vi "数据查询_数据查询.vi"() -> ()   [LabVIEW 2016, in "数据查询.lvlib"]
uses:
  System.Windows.Forms
  <vilib>/Utility/miscctls.llb/LVPointTypeDef.ctl
  <userlib>/_OpenG.lib/array/array.llb/Sort 2D Array (String)__ogtk.vi
  <vilib>/ptbypt/NI_PtbyPt.lvlib
panel:
  in  "数据类型":string(combo)="N"
  out "columns":string[](array[string])
  out "表格":string[][](table)
  in  "剔除异常数据":bool=TRUE
  in  "WebBrowser":refnum<k24>(container)
  in  "列表框":i32(listbox)
  in  "导出":bool
  in  "测量模式":string(combo)="全部数据"
  out "选中数据表":string
  in  "查询":bool
  in  "结束日期":string="2050/01/01"
  in  "起始日期":string="2010/01/01"
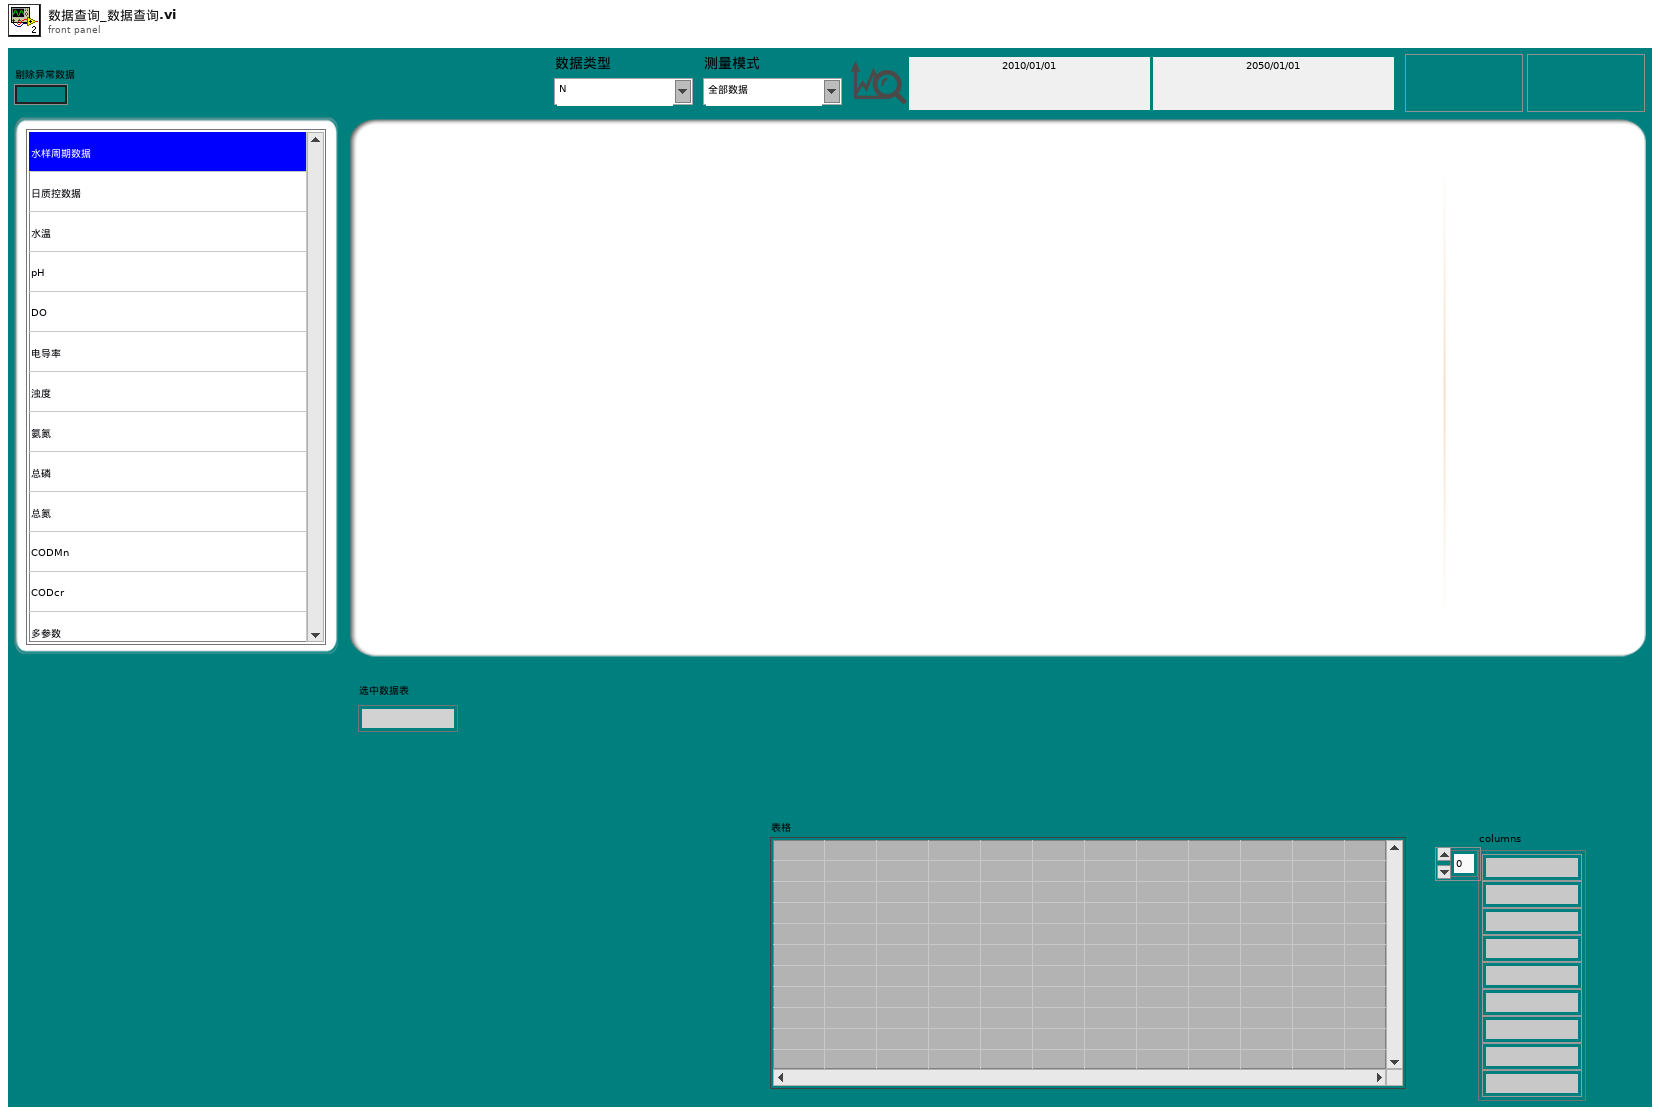
[diagram p1: front panel]
types:
  T1 = typedef "LVPointTypeDef.ctl" = cluster{"Horizontal":i16, "Vertical":i16}
  T2 = typedef "LVDateTimeRec.ctl" = cluster{"秒数的小数部分":dbl, "秒":i32, "分":i32, "时":i32, "日":i32, "月":i32, "年":i32, "天数（周）":i32, "天数（年）":i32, "DST":i32}
  T3 = typedef "数据查询菜单.xctl/数据 1.ctl" = enum32{"数据查询", "仪器数据", "仪器日志", "报警信息", "校准日志"}
  T4 = enum8{"Enabled", "Disabled", "Disabled and Grayed Out"}
  T5 = typedef "数据库类型.ctl" = enum16{"Access", "SQLite"}
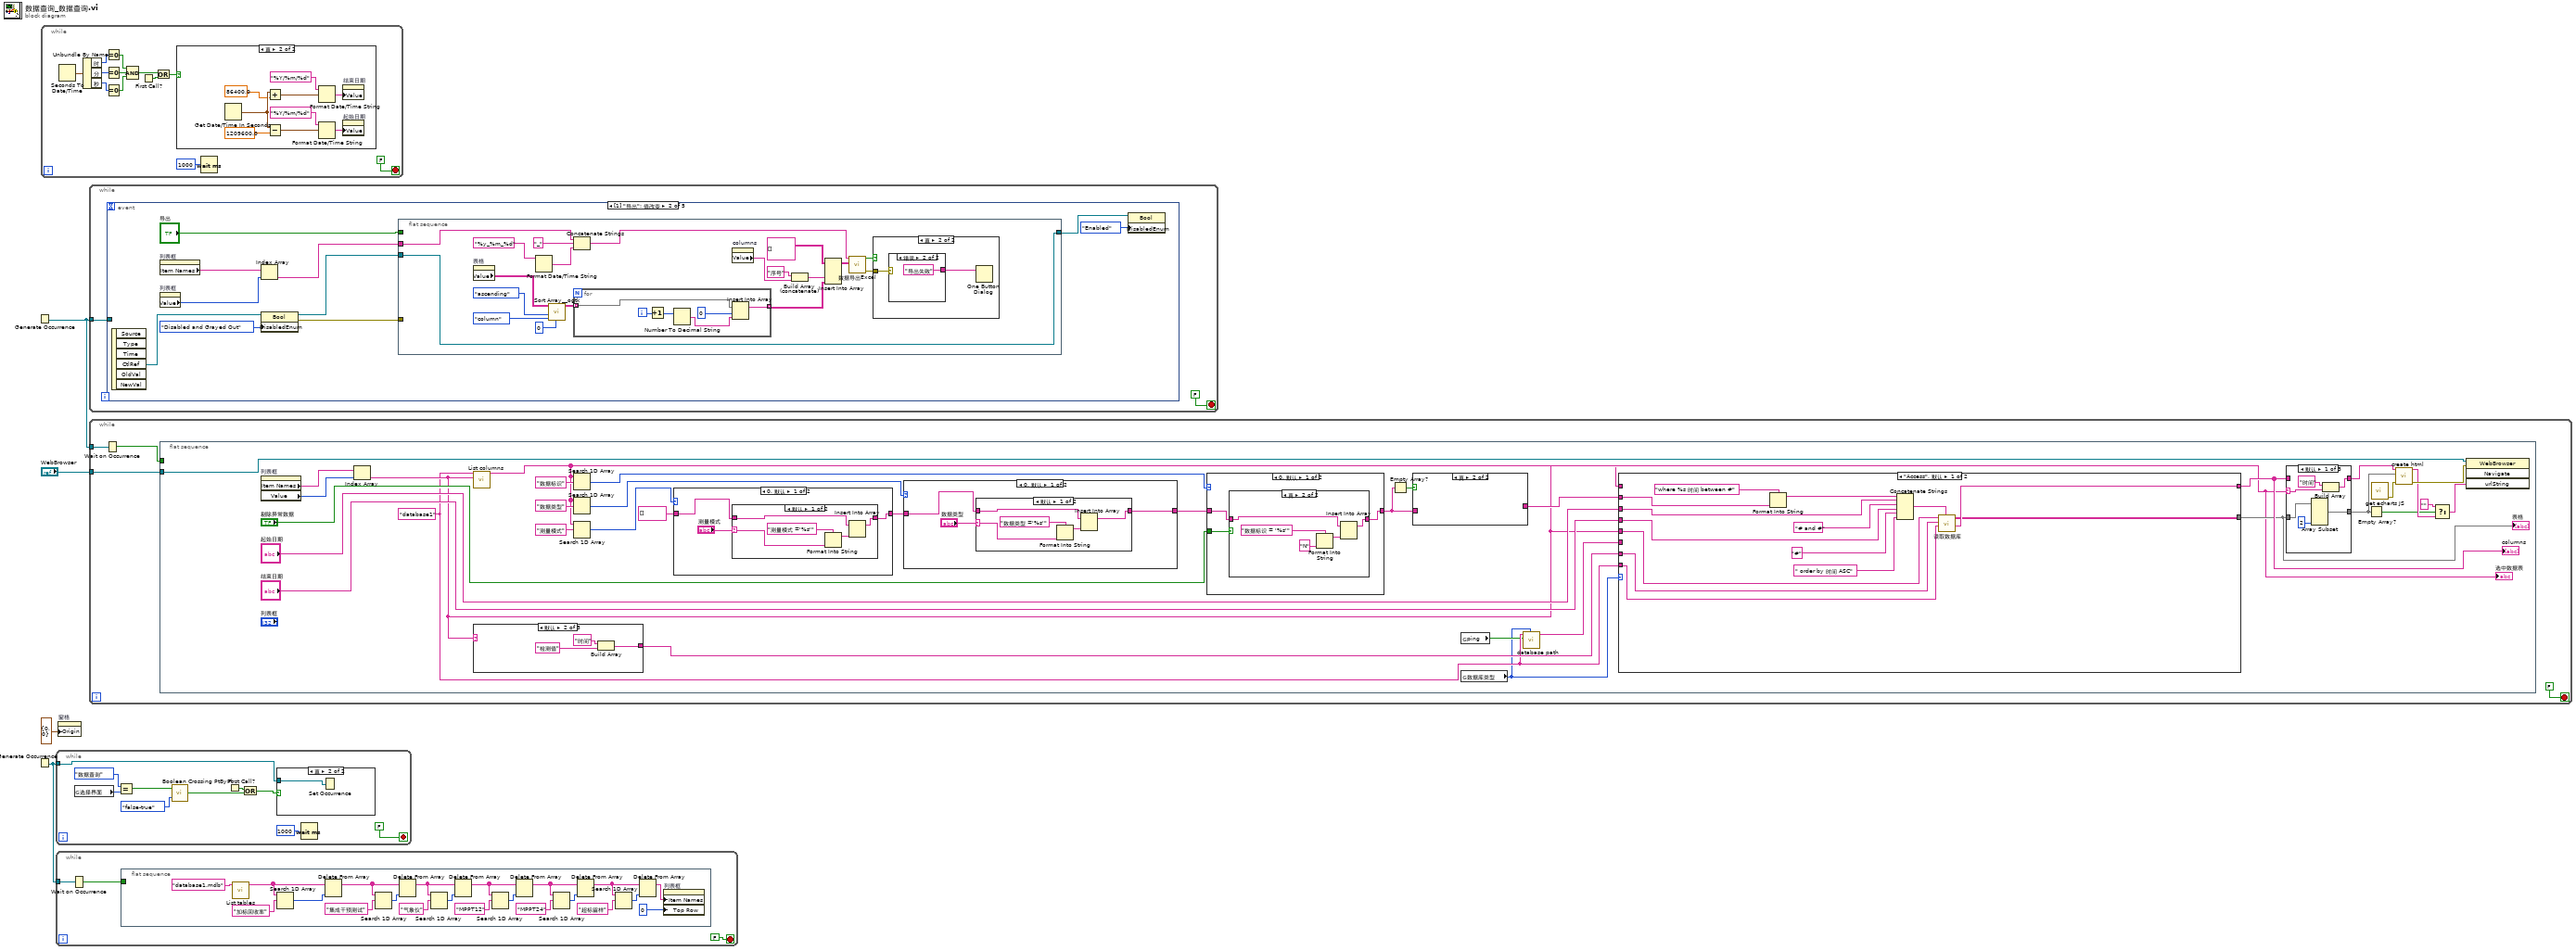
[diagram p0: block diagram]
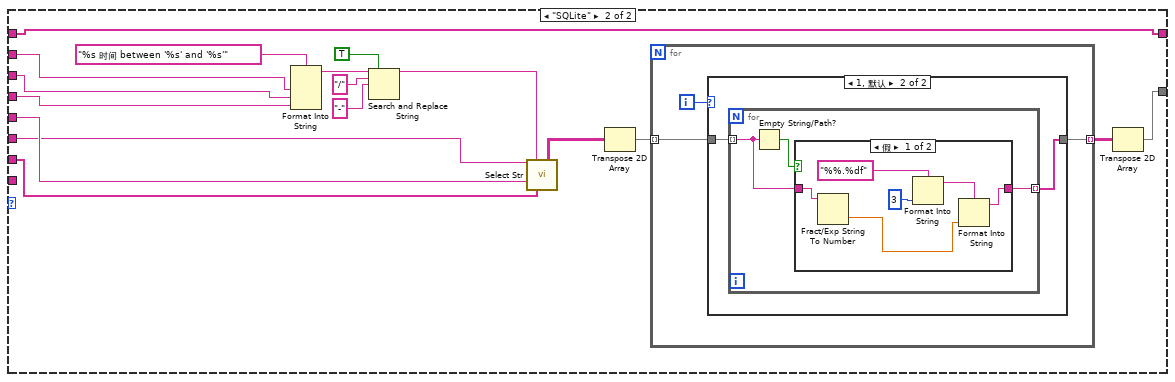
[diagram p3: hidden frame]
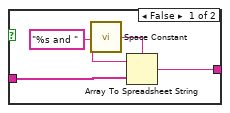
[diagram p6: hidden frame]
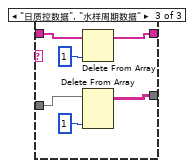
[diagram p14: hidden frame]
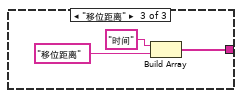
[diagram p16: hidden frame]
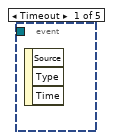
[diagram p18: hidden frame]
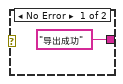
[diagram p20: hidden frame]
diagram:
  n1 = Generate Occurrence() -> (w3:refnum<k4>)
  n2 = Generate Occurrence() -> (w1:refnum<k4>)
  n3 = while {
    stop <- FALSE stop-if-true
    n4 = Seconds To Date/Time() -> (date time rec=w16:T2)  [unwired: 2 in]
    n5 = Unbundle By Name(w16) -> ("时"=w15:i32, "分"=w14:i32, "秒"=w13:i32)
    n6 = Equal To 0?(x=w15) -> (x = 0?=w12:bool)
    n7 = Equal To 0?(x=w14) -> (x = 0?=w11:bool)
    n8 = Equal To 0?(x=w13) -> (x = 0?=w10:bool)
    n9 = Compound Arithmetic op=AND ("复合运算")(w12, w11, w10) -> (w7:bool)
    n10 = First Call?() -> (First Call?: T/F=w5:bool)
    n11 = Or(x=w7, y=w5) -> (x .or. y?=w6:bool)
    n12 = case shown="真" w6 {
      frame False {
      }
      frame True {
        n13 = Get Date/Time In Seconds() -> (seconds since 1Jan1904=w21:timestamp)
        n14 = Add(x=w21, y=86400.0) -> (x+y=w19:timestamp)
        n15 = Subtract(x=w21, y=1209600.0) -> (x-y=w22:timestamp)
        n16 = Format Date/Time String(time format string (%c)="%Y/%m/%d" ("时间格式字符串(%c)"), seconds (now)=w19) -> (date/time string=w18:string)  [unwired: 1 in]
        n17 = Format Date/Time String(time format string (%c)="%Y/%m/%d" ("时间格式字符串(%c)"), seconds (now)=w22) -> (date/time string=w24:string)  [unwired: 1 in]
        n18 = property on="结束日期" class="Str"("Value"=w18) -> ()  [unwired: 2 in, 2 out]
        n19 = property on="起始日期" class="Str"("Value"=w24) -> ()  [unwired: 2 in, 2 out]
      }
    }
    n20 = Wait (ms)(milliseconds to wait=u32 1000 ("等待时间（毫秒）")) -> ()  [unwired: 1 out]
  }
  n21 = while {
    tunnel: w1 -> [w33]
    stop <- FALSE stop-if-true
    n22 = global read "全局变量.vi" "选择界面"() -> (w32:T3)
    n23 = Equal?(x=数据_1."数据查询", y=w32) -> (x = y?=w30:bool)
    n24 = call <vilib>:"Boolean Crossing PtByPt.vi"("direction"=enum16{"either", "false-true", "true-false"}."false-true", "input"=w30) -> ("crossing"=w28:bool)  [unwired: 1 in]
    n25 = First Call?() -> (First Call?: T/F=w26:bool)
    n26 = Or(x=w26, y=w28) -> (x .or. y?=w27:bool)
    n27 = case shown="真" w27 {
      tunnel: w33 -> [_ w36]
      frame False {
      }
      frame True {
        n28 = Set Occurrence(w36) -> ()
      }
    }
    n29 = Wait (ms)(milliseconds to wait=u32 1000 ("等待时间（毫秒）")) -> ()  [unwired: 1 out]
  }
  n30 = while {
    tunnel: w1 -> [w38]
    stop <- FALSE stop-if-true
    n31 = Wait on Occurrence(2:w38) -> (0:w37:bool)  [unwired: 2 in]
    n32 = flat-sequence {
      tunnel: w37 -> [_]
      frame #0 {
        n33 = call "List tables.vi"("database"="database1.mdb") -> ("tables"=w44:string[])  [unwired: 9 in, 1 out]
        n34 = Search 1D Array(1D array=w44, element="加标回收率" ("元素")) -> (index of element=w45:i32)  [unwired: 1 in]
        n35 = Delete From Array(array=w44, index=w45) -> (array with subset deleted=w47:string[])  [unwired: 1 in, 1 out]
        n36 = Search 1D Array(1D array=w47, element="集成干预测试" ("元素")) -> (index of element=w46:i32)  [unwired: 1 in]
        n37 = Delete From Array(array=w47, index=w46) -> (array with subset deleted=w50:string[])  [unwired: 1 in, 1 out]
        n38 = Search 1D Array(1D array=w50, element="气象仪" ("元素")) -> (index of element=w48:i32)  [unwired: 1 in]
        n39 = Delete From Array(array=w50, index=w48) -> (array with subset deleted=w53:string[])  [unwired: 1 in, 1 out]
        n40 = Search 1D Array(1D array=w53, element="MPPT12" ("元素")) -> (index of element=w52:i32)  [unwired: 1 in]
        n41 = Delete From Array(array=w53, index=w52) -> (array with subset deleted=w56:string[])  [unwired: 1 in, 1 out]
        n42 = Search 1D Array(1D array=w56, element="MPPT24" ("元素")) -> (index of element=w54:i32)  [unwired: 1 in]
        n43 = Delete From Array(array=w56, index=w54) -> (array with subset deleted=w57:string[])  [unwired: 1 in, 1 out]
        n44 = Search 1D Array(1D array=w57, element="超标留样" ("元素")) -> (index of element=w59:i32)  [unwired: 1 in]
        n45 = Delete From Array(array=w57, index=w59) -> (array with subset deleted=w60:string[])  [unwired: 1 in, 1 out]
        n46 = property on="列表框" class="LstBox (严格)"("Item Names"=w60, "Top Row"=0 ("顶行")) -> ()  [unwired: 2 in, 2 out]
      }
    }
  }
  n47 = property on="窗格" class="Pane"("Origin"=T1 {"Horizontal"=0, "Vertical"=0} ("原点")) -> ()  [unwired: 2 in, 2 out]
  n48 = while {
    tunnel: w3 -> [w61]
    stop <- FALSE stop-if-true
    n49 = event shown="[1] \"导出\": 值改变" {
      selector: _ -> [_ _ _ _ _]
      dyn-events: _ -> [_ _ _ _ _]
      timeout: _ -> [_ _ _ _ _]
      tunnel: w61 -> [_ _ _ w106 w107]
      event Timeout {
        n50 = event-data() -> ()  [unwired: 1 in, 3 out]
      }
      event "导出": Value Change {
        n51 = event-data() -> ("CtlRef"=w72:refnum<vi>)  [unwired: 1 in, 5 out]
        n52 = property on="列表框" class="LstBox (严格)"() -> ("Item Names"=w65:string[])  [unwired: 2 in, 2 out]
        n53 = property on="列表框" class="LstBox (严格)"() -> ("Value"=w64:i32)  [unwired: 2 in, 2 out]
        n54 = Index Array(array=w65, index=w64) -> (element=w63:string)
        n55 = property class="Bool"(reference=w72, "DisabledEnum"=T4."Disabled and Grayed Out" ("禁用")) -> (reference out=w69:refnum<vi>, error out=w70:errorcluster)  [unwired: 1 in]
        n56 = flat-sequence {
          tunnel: w70 -> [_]
          tunnel: [w88] -> w68
          tunnel: w69 -> [w88]
          tunnel: "导出" -> [_]
          tunnel: w63 -> [w78]
          frame #0 {
            n57 = property on="表格" class="Tbl (严格)"() -> ("Value"=w74:string[][])  [unwired: 2 in, 2 out]
            n58 = Format Date/Time String(time format string (%c)="%y_%m_%d" ("时间格式字符串(%c)")) -> (date/time string=w85:string)  [unwired: 2 in]
            n59 = call-poly <userlib>:"Sort Array__ogtk.vi"("Column/Row to Sort By"=u32 0, "Sort By in"=enum16{"row", "column"}."column", "Order"=enum16{"ascending", "descending"}."ascending", "Array in"=w74) -> ("Sorted Array out"=w82:string[][])  [unwired: 4 in, 3 out]
            n60 = Concatenate Strings(w78, "_" ("字符串"), w85) -> (w83:string)
            n61 = for {
              tunnel: w82 -> [w100] mode=indexing
              tunnel: [w99] -> w75 mode=indexing
              i -> [w101]
              n62 = Increment(x=w101) -> (x+1=w97:i32)
              n63 = Number To Decimal String(number=w97) -> (decimal integer string=w96:string)  [unwired: 1 in]
              n64 = Insert Into Array(array=w100, index=0 ("索引"), new element=w96) -> (w99:string[])
            }
            n65 = property on="columns" class="Arr (严格)"() -> ("Value"=w73:string[])  [unwired: 2 in, 2 out]
            n66 = Build Array (concatenate)("序号" ("新元素/子数组"), w73) -> (w76:string[])
            n67 = Insert Into Array(array=string[][] [], new element #1=w76, new element #2=w75) -> (w81:string[][])  [unwired: 2 in]
            n68 = call "数据导出Excel.vi"("text data"=w81, "default name"=w83) -> ("error out"=w80:errorcluster, "布尔"=w79:bool)  [unwired: 8 in]
            n69 = case shown="真" w79 {
              tunnel: w80 -> [_ w93]
              frame False {
              }
              frame True {
                n70 = case shown="错误" w93 {
                  tunnel: ["导出成功" ("消息") "导出失败" ("消息")] -> w92
                  frame No Error {
                  }
                  frame Error {
                  }
                }
                n71 = One Button Dialog(message=w92) -> ()  [unwired: 1 in, 1 out]
              }
            }
          }
        }
        n72 = property class="Bool"(reference=w68, "DisabledEnum"=T4."Enabled" ("禁用")) -> ()  [unwired: 1 in, 2 out]
      }
      event "起始日期", "结束日期": Mouse Down {
        n73 = event-data() -> ("CtlRef"=w105:refnum<vi>)  [unwired: 1 in, 7 out]
        n74 = property class="Str"(reference=w105) -> (reference out=w103:refnum<vi>, "Value"=w104:string)  [unwired: 1 in, 1 out]
        n75 = call "日期键盘.vi"("原值"=w104) -> ("x+y"=w102:string)  [unwired: 10 in]
        n76 = property class="Str"(reference=w103, "Val(Sgnl)"=w102) -> ()  [unwired: 1 in, 2 out]
      }
      event "查询", "起始日期", "结束日期", "测量模式", "剔除异常数据", "数据类型": Value Change {
        n77 = event-data() -> ()  [unwired: 1 in, 6 out]
        n78 = Set Occurrence(w106) -> ()
      }
      event "列表框": Value Change; "列表框": Mouse Down {
        n79 = event-data() -> ()  [unwired: 1 in, 4 out]
        n80 = flat-sequence {
          tunnel: [w109] -> w108
          tunnel: w107 -> [w109]
          tunnel: w108 -> [w112]
          frame #0 {
            n81 = property on="数据类型" class="CmbBox"("Value"="N" ("数据类型")) -> ()  [unwired: 2 in, 2 out]
            n82 = property on="测量模式" class="CmbBox"("Value"="全部数据" ("测量模式")) -> ()  [unwired: 2 in, 2 out]
          }
          frame #1 {
            n83 = Set Occurrence(w112) -> ()
          }
        }
      }
    }
  }
  n84 = while {
    tunnel: w3 -> [w115]
    tunnel: "WebBrowser" -> [w113]
    stop <- FALSE stop-if-true
    n85 = Wait on Occurrence(2:w115) -> (0:w114:bool)  [unwired: 2 in]
    n86 = flat-sequence {
      tunnel: w114 -> [_]
      tunnel: w113 -> [w149]
      frame #0 {
        w119 = "database1" ("database")
        n87 = property on="列表框" class="LstBox (严格)"() -> ("Item Names"=w141:string[], "Value"=w140:i32)  [unwired: 2 in, 2 out]
        n88 = Index Array(array=w141, index=w140) -> (element=w132:string)
        "选中数据表" <- w132
        n89 = call "List columns.vi"("table"=w132, "database"=w119) -> ("columns"=w121:string[])  [unwired: 8 in, 1 out]
        n90 = case shown="默认" w132 {
          tunnel: [_ w247 w250] -> w143
          frame "多参数", "环境参数", "日质控数据", "水样周期数据" {
          }
          frame Default {
            n91 = Build Array("时间", "检测值") -> (w247:string[])
          }
          frame "移位距离" {
            n92 = Build Array("时间", "移位距离") -> (w250:string[])
          }
        }
        n93 = Search 1D Array(1D array=w121, element="数据标识" ("元素")) -> (index of element=w124:i32)  [unwired: 1 in]
        n94 = Search 1D Array(1D array=w121, element="数据类型" ("元素")) -> (index of element=w125:i32)  [unwired: 1 in]
        n95 = Search 1D Array(1D array=w121, element="测量模式" ("元素")) -> (index of element=w127:i32)  [unwired: 1 in]
        n96 = case shown="0, 默认" w127 {
          tunnel: string[] [] -> [w225 w232]
          tunnel: [w223 w232] -> w126
          frame 0, Default {
            n97 = case shown="默认" "测量模式" {
              selector: "测量模式" -> [w226 _]
              tunnel: w225 -> [w229 w231]
              tunnel: [w227 w231] -> w223
              frame Default {
                n98 = Format Into String(format string="测量模式 ='%s'" ("condition"), w226) -> (resulting string=w228:string)  [unwired: 2 in, 1 out]
                n99 = Insert Into Array(array=w229, new element=w228) -> (w227:string[])  [unwired: 1 in]
              }
              frame "全部数据" {
              }
            }
          }
          frame -1 {
          }
        }
        n100 = case shown="0, 默认" w125 {
          tunnel: [w214 w222] -> w128
          tunnel: w126 -> [w213 w222]
          frame 0, Default {
            n101 = case shown="默认" "数据类型" {
              selector: "数据类型" -> [w216 _]
              tunnel: w213 -> [w219 w221]
              tunnel: [w217 w221] -> w214
              frame Default {
                n102 = Format Into String(format string="数据类型 ='%s'" ("condition"), w216) -> (resulting string=w218:string)  [unwired: 2 in, 1 out]
                n103 = Insert Into Array(array=w219, new element=w218) -> (w217:string[])  [unwired: 1 in]
              }
              frame "全部数据" {
              }
            }
          }
          frame -1 {
          }
        }
        n104 = case shown="0, 默认" w124 {
          tunnel: "剔除异常数据" -> [w205 _]
          tunnel: [w204 w212] -> w123
          tunnel: w128 -> [w203 w212]
          frame 0, Default {
            n105 = case shown="真" w205 {
              tunnel: w203 -> [w206 w211]
              tunnel: [w206 w210] -> w204
              frame False {
              }
              frame True {
                n106 = Format Into String(format string="数据标识 = '%s'" ("condition"), "N" ("String")) -> (resulting string=w207:string)  [unwired: 2 in, 1 out]
                n107 = Insert Into Array(array=w211, new element=w207) -> (w210:string[])  [unwired: 1 in]
              }
            }
          }
          frame -1 {
          }
        }
        n108 = Empty Array?(array=w123) -> (empty?=w122:bool)
        n109 = case shown="真" w122 {
          tunnel: [w202 _] -> w133
          tunnel: w123 -> [w199 _]
          frame False {
            n110 = call <vilib>:"Space Constant.vi"() -> ("String"=w201:string)
            n111 = Array To Spreadsheet String(delimiter (Tab)=w201, array=w199, 3:"%s and " ("格式字符串")) -> (spreadsheet string=w202:string)
          }
          frame True {
          }
        }
        n112 = global read "全局变量.vi" "ping"() -> (w118:bool)
        n113 = global read "全局变量.vi" "数据库类型"() -> (w117:T5)
        n114 = call "database path.vi"("数据库类型"=w117, "ping"=w118, "database"=w119) -> ("Path out"=w120:string)  [unwired: 8 in]
        n115 = case shown="\"Access\", 默认" w117 {
          tunnel: "结束日期" -> [w161 w173]
          tunnel: "起始日期" -> [w160 w174]
          tunnel: [w159 w171] -> w146
          tunnel: [w158 w172] -> w144
          tunnel: w143 -> [w157 w167]
          tunnel: w133 -> [w156 w175]
          tunnel: w132 -> [w153 w168]
          tunnel: w121 -> [_ w171]
          tunnel: w120 -> [_ w166]
          tunnel: w119 -> [w152 _]
          frame "Access", Default {
            n116 = Format Into String(format string="where %s 时间 between #" ("condition"), w156) -> (resulting string=w154:string)  [unwired: 2 in, 1 out]
            n117 = Concatenate Strings(w154, w160, "# and #" ("condition"), w161, "#" ("condition"), " order by 时间 ASC" ("字符串")) -> (w165:string)
            n118 = call "读取数据库.vi"("condition"=w165, "database"=w152, "显示项"=w157, "组合框"=w153) -> ("columns"=w159:string[], "表格"=w158:string[][])  [unwired: 4 in, 2 out]
          }
          frame "SQLite" {
            n119 = Format Into String(format string="%s 时间 between '%s' and '%s'" ("格式字符串"), w175, w174, w173) -> (resulting string=w178:string)  [unwired: 2 in, 1 out]
            n120 = Search and Replace String(replace all?=TRUE ("替换全部？(F)"), input string=w178, search string="/" ("搜索字符串"), replace string="-" ("替换字符串(\"\")")) -> (result string=w170:string)  [unwired: 4 in, 3 out]
            n121 = call "Select Str.vi"("DB Path"=w166, "Where Clause"=w170, "Tables Name"=w168, "Columns"=w167) -> ("Results"=w169:string[][])  [unwired: 8 in, 3 out]
            n122 = Transpose 2D Array(2D array=w169) -> (transposed array=w177:string[][])
            n123 = for {
              tunnel: w177 -> [w185] mode=indexing
              tunnel: [w184] -> w176 mode=indexing
              i -> [w183]
              n124 = case shown="1, 默认" w183 {
                tunnel: w185 -> [w186 w188]
                tunnel: [w186 w187] -> w184
                frame 0 {
                }
                frame 1, Default {
                  n125 = for {
                    tunnel: w188 -> [w190] mode=indexing
                    tunnel: [w191] -> w187 mode=indexing
                    n126 = Empty String/Path?(string/path=w190) -> (empty?=w189:bool)
                    n127 = case shown="假" w189 {
                      tunnel: [w195 w198] -> w191
                      tunnel: w190 -> [w192 w198]
                      frame False {
                        n128 = Fract/Exp String To Number(string=w192) -> (number=w194:dbl)  [unwired: 3 in, 1 out]
                        n129 = Format Into String(format string="%%.%df" ("格式字符串"), 3 ("输入 1")) -> (resulting string=w197:string)  [unwired: 2 in, 1 out]
                        n130 = Format Into String(format string=w197, w194) -> (resulting string=w195:string)  [unwired: 2 in, 1 out]
                      }
                      frame True {
                      }
                    }
                  }
                }
              }
            }
            n131 = Transpose 2D Array(2D array=w176) -> (transposed array=w172:string[][])
          }
        }
        "表格" <- w144
        "columns" <- w146
        n132 = case shown="默认" w132 {
          selector: w132 -> [w235 _ _]
          tunnel: w146 -> [_ w240 w246]
          tunnel: [w234 w240 w245] -> w145
          tunnel: w144 -> [w238 w239 w243]
          tunnel: [w237 w239 w242] -> w136
          frame Default {
            n133 = Array Subset(array=w238, length (col)=2 ("长度")) -> (w237:string[][])  [unwired: 3 in]
            n134 = Build Array("时间", w235) -> (w234:string[])
          }
          frame "多参数", "环境参数" {
          }
          frame "日质控数据", "水样周期数据" {
            n135 = Delete From Array(array=w246, index=1 ("索引")) -> (array with subset deleted=w245:string[])  [unwired: 1 in, 1 out]
            n136 = Delete From Array(array=w243, index (col)=1 ("禁用的索引 (列)")) -> (array with subset deleted=w242:string[][])  [unwired: 2 in, 1 out]
          }
        }
        n137 = Empty Array?(array=w136) -> (empty?=w135:bool)
        n138 = call "get echarts JS.vi"() -> ("error out"=w148:errorcluster)  [unwired: 11 in]
        n139 = call "create html.vi"("error in (no error)"=w148, "data"=w136, "columns"=w145) -> ("error out"=w147:errorcluster, "url"=w139:string)  [unwired: 7 in]
        n140 = Select(t="", s=w135, f=w139) -> (s? t:f=w138:string)
        n141 = invoke class="WebBrowser" method="Navigate"(reference=w149, error in=w147, "urlString"=w138) -> ()  [unwired: 1 in, 4 out]
      }
    }
  }
